vi "Unit test-Logging queue warning windows.vi"() -> ()   [LabVIEW 2017]
panel:
  in  "Slide":i32(slide) scale=0.0..25000.0
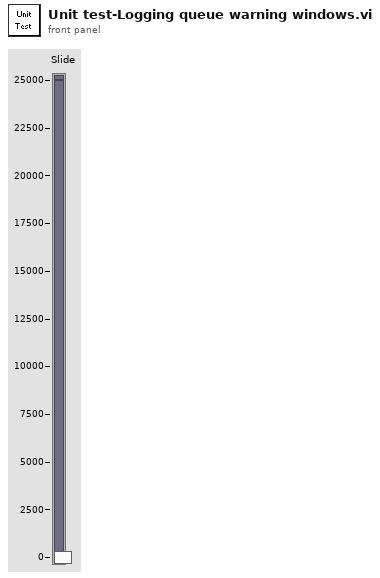
[diagram p1: front panel]
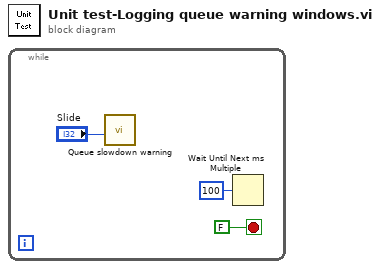
[diagram p0: block diagram]
diagram:
  n1 = while {
    stop <- FALSE stop-if-true
    n2 = call "Queue slowdown warning.vi"("# elements in queue in"="Slide") -> ()  [unwired: 11 in]
    n3 = Wait Until Next ms Multiple(millisecond multiple=u32 100) -> ()  [unwired: 1 out]
  }
